vi "Find Closest SCM Microphone.vi"(5 "Source Polar\nCoordinates":cluster{"r":dbl, "theta":dbl}, 9 "Microphone Coordinates (cm, rad)":cluster{"r":dbl, "theta":dbl}[](array[cluster])) -> (6 "Closest Microphone Index":i32, 10 "Closest Microphone Distance (cm)":dbl)   [LabVIEW 2013, in "Breakdown Acoustics Controls.lvlib"]
uses:
  Breakdown Acoustics Controls.lvlib
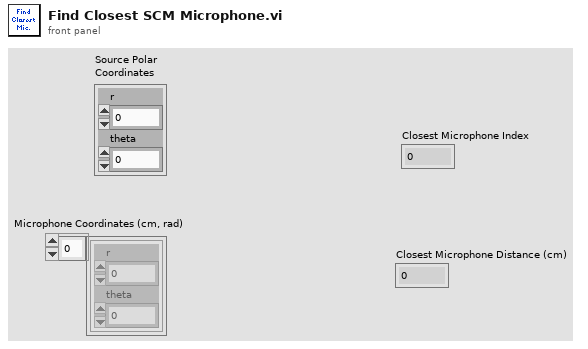
[diagram p1: front panel]
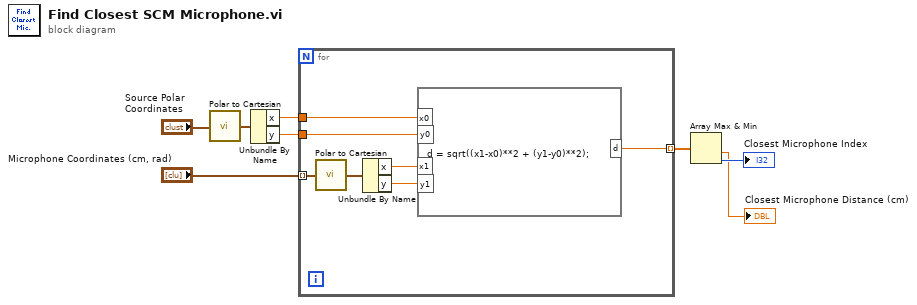
[diagram p0: block diagram]
diagram:
  n1 = call "Polar to Cartesian.vi"("Polar\nCoordinates"="Source Polar\nCoordinates") -> ("Cartesian\nCoordinates"=w6:cluster{"x":dbl, "y":dbl})  [unwired: 4 in]
  n2 = Unbundle By Name(w6) -> ("x"=w5:dbl, "y"=w4:dbl)
  n3 = for {
    tunnel: "Microphone Coordinates (cm, rad)" -> [w15] mode=indexing
    tunnel: w5 -> [w14]
    tunnel: w4 -> [w13]
    tunnel: [w9] -> w3 mode=indexing
    n4 = call "Polar to Cartesian.vi"("Polar\nCoordinates"=w15) -> ("Cartesian\nCoordinates"=w12:cluster{"x":dbl, "y":dbl})  [unwired: 4 in]
    n5 = Unbundle By Name(w12) -> ("x"=w11:dbl, "y"=w10:dbl)
    n6 = formula code="d = sqrt((x1-x0)**2 + (y1-y0)**2);"("x0"=w14, "y0"=w13, "x1"=w11, "y1"=w10) -> ("d"=w9:dbl)
  }
  n7 = Array Max & Min(array=w3) -> (min value=→"Closest Microphone Distance (cm)":dbl, min index (indices)=→"Closest Microphone Index":i32)  [unwired: 2 out]
